vi "GoToHeightController.vi"(6 "Command Timing":cluster{"Start Time (ms)":u32, "Iterations":i32}, 10 "Position":i32, 11 "Setpoints":T2) -> (0 "Done":bool, 1 "DemandType":T3(ring), 2 "Output":i32, 3 "Control Mode":T4 items=["PercentOutput"=0, "Position"=1, "Velocity"=2, "Current"=3, "Follower"=5, "MotionProfile"=6, "MotionMagic"=7, "MotionProfileArc"=10, "Disabled"=15], 4 "Delay":dbl)   [LabVIEW 2018]
uses:
  <vilib>/Rock Robotics/WPI/ThirdParty/Phoenix-LabVIEW/Motor Controller/Controls/CTRE_Phoenix_MotorControl_ControlMode.ctl
  Implementation/Arm Operations.ctl
  Configuration/Constants.vi
  Drive/Implementation/Drive Published Globals.vi
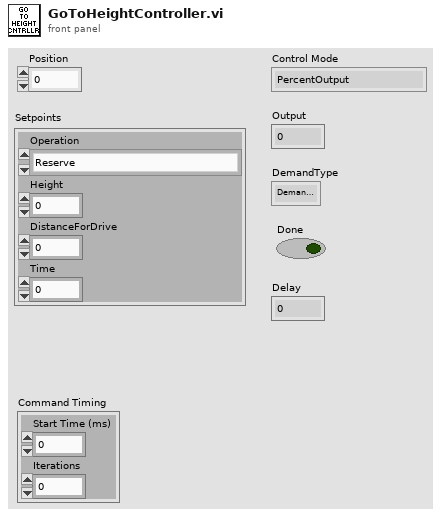
[diagram p1: front panel]
types:
  T1 = typedef "Arm Operations.ctl" = enum16{"Reserve", "Read Current", "Immediate", "RaiseForTime", "GoToHeight", "StayAtHeight", "RaiseAfterTime", "RaiseAfterDriveAtDistance"}
  T2 = cluster{"Operation":T1, "Height":dbl, "DistanceForDrive":dbl, "Time":dbl}
  T3 = enum16{"DemandType_Neutral", "DemandType_AuxPID", "DemandType_ArbitraryFeedForward"}
  T4 = typedef "CTRE_Phoenix_MotorControl_ControlMode.ctl" = u16
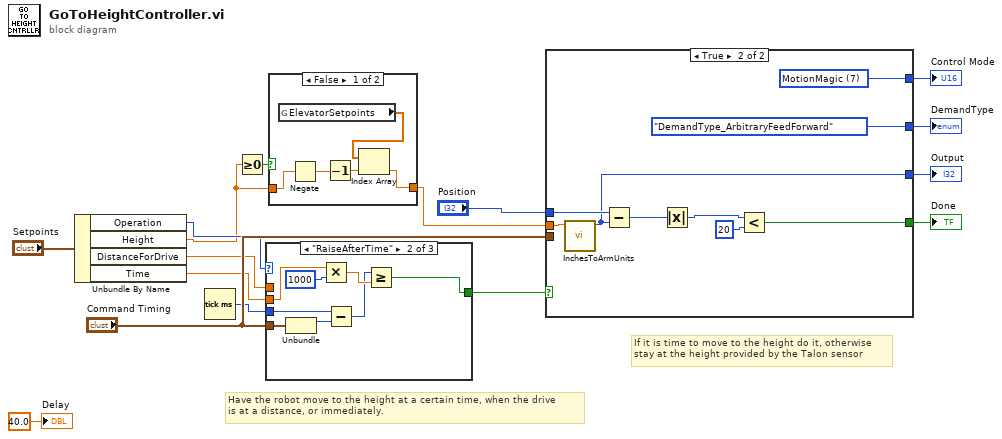
[diagram p0: block diagram]
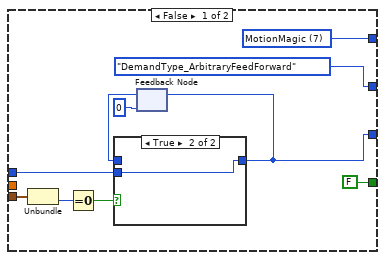
[diagram p3: hidden frame]
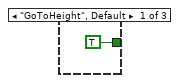
[diagram p5: hidden frame]
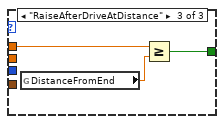
[diagram p6: hidden frame]
diagram:
  # "If it is time to move to the height do it, otherwise\nstay at the height provided by the Talon sensor"
  # "Have the robot move to the height at a certain time, when the drive\nis at a distance, or immediately."
  n1 = Unbundle By Name("Setpoints") -> ("Operation"=w6:T1, "Height"=w2:dbl, "DistanceForDrive"=w5:dbl, "Time"=w4:dbl)
  n2 = Tick Count (ms)() -> (millisecond timer value=w8:u32)
  n3 = Greater Or Equal To 0?(x=w2) -> (x >= 0?=w3:bool)
  n4 = case shown="\"RaiseAfterTime\"" w6 {
    tunnel: [TRUE w18 w27] -> w9
    tunnel: w8 -> [_ w22 _]
    tunnel: "Command Timing" -> [_ w23 _]
    tunnel: w4 -> [_ w25 _]
    tunnel: w5 -> [_ _ w28]
    frame "GoToHeight", Default {
    }
    frame "RaiseAfterTime" {
      n5 = Unbundle(w23) -> ("Start Time (ms)"=w21:u32)  [unwired: 1 out]
      n6 = Multiply(x=w25, y=1000) -> (x*y=w20:dbl)
      n7 = Subtract(x=w22, y=w21) -> (x-y=w19:u32)
      n8 = Greater Or Equal?(x=w19, y=w20) -> (x >= y?=w18:bool)
    }
    frame "RaiseAfterDriveAtDistance" {
      n9 = global read "Drive Published Globals.vi" "DistanceFromEnd"() -> (w26:dbl)
      n10 = Greater Or Equal?(x=w28, y=w26) -> (x >= y?=w27:bool)
    }
  }
  n11 = case shown="False" w3 {
    tunnel: [w29 w34] -> w1
    tunnel: w2 -> [w31 w34]
    frame False {
      n12 = global read "Constants.vi" "ElevatorSetpoints"() -> (w30:dbl[])
      n13 = Negate(x=w31) -> (-x=w32:dbl)
      n14 = Decrement(x=w32) -> (x-1=w33:dbl)
      n15 = Index Array(array=w30, index=w33) -> (element=w29:dbl)
    }
    frame True {
    }
  }
  n16 = case shown="True" w9 {
    tunnel: [FALSE w48] -> w11
    tunnel: [T3."DemandType_ArbitraryFeedForward" ("DemandType") T3."DemandType_ArbitraryFeedForward" ("DemandType")] -> w12
    tunnel: [w38 w53] -> w13
    tunnel: "Position" -> [w40 w54]
    tunnel: [w43 w52] -> w15
    tunnel: "Command Timing" -> [w41 _]
    tunnel: w1 -> [_ w47]
    frame False {
      w43 = T4 7 items=["PercentOutput"=0, "Position"=1, "Velocity"=2, "Current"=3, "Follower"=5, "MotionProfile"=6, "MotionMagic"=7, "MotionProfileArc"=10, "Disabled"=15] ("Control Mode")
      n17 = Unbundle(w41) -> ("Iterations"=w35:i32)  [unwired: 1 out]
      n18 = Equal To 0?(x=w35) -> (x = 0?=w36:bool)
      n19 = feedback #1(0 ("Position")) -> (w39:i32)
      n20 = case shown="True" w36 {
        tunnel: [w45 w46] -> w38
        tunnel: w40 -> [_ w46]
        tunnel: w39 -> [w45 _]
        frame False {
        }
        frame True {
        }
      }
      n21 = feedback-in #1(w38) -> ()
    }
    frame True {
      w52 = T4 7 items=["PercentOutput"=0, "Position"=1, "Velocity"=2, "Current"=3, "Follower"=5, "MotionProfile"=6, "MotionMagic"=7, "MotionProfileArc"=10, "Disabled"=15] ("Control Mode")
      n22 = call "InchesToArmUnits.vi"("Inches"=w47) -> ("Sensor Units"=w53:i32)  [unwired: 10 in]
      n23 = Subtract(x=w54, y=w53) -> (x-y=w51:i32)
      n24 = Absolute Value(x=w51) -> (abs(x)=w50:i32)
      n25 = Less?(x=w50, y=20) -> (x < y?=w48:bool)
    }
  }
  "Control Mode" <- w15
  "Output" <- w13
  "DemandType" <- w12
  "Done" <- w11
  "Delay" <- 40.0 ("Infinite")
